vi "MultiChannelBeta3.vi"() -> ()   [LabVIEW 2014]
panel:
  in  "File Path Control":path
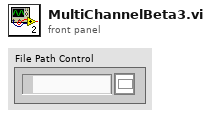
[diagram p1: front panel]
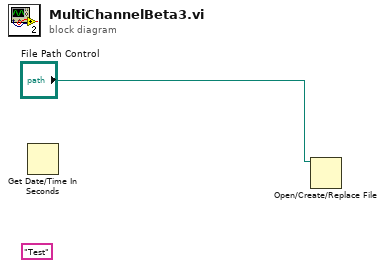
[diagram p0: block diagram]
diagram:
  (unwired) "Test"
  n1 = Get Date/Time In Seconds() -> ()  [unwired: 1 out]
  n2 = Open/Create/Replace File(file path (use dialog)="File Path Control") -> ()  [unwired: 5 in, 3 out]
